vi "PT3_Create.vi"(5 "Save pt3":bool=TRUE, 7 "overwrite existing":bool, 8 "error in":errorcluster, 9 "Comment":string, 10 "pt3 header in":T1={"Comment"="", "RangeNo"=0, "Offset"=0, "AcquisitionTime (ms)"=0, "HardwareSerial"=0, "SyncDivider"=0, "Resolution (ns)"=0.0, "CFD Settings"={"Ch0 Level"=150, "Ch0 ZeroX"=10, "Ch1 Level"=50, "Ch1 ZeroX"=10}, "InpRate0"=0, "InpRate1"=0}, 11 "File Path":path) -> (0 "error out":errorcluster, 3 "refnum out":refnum<file>)   [LabVIEW 8.6]
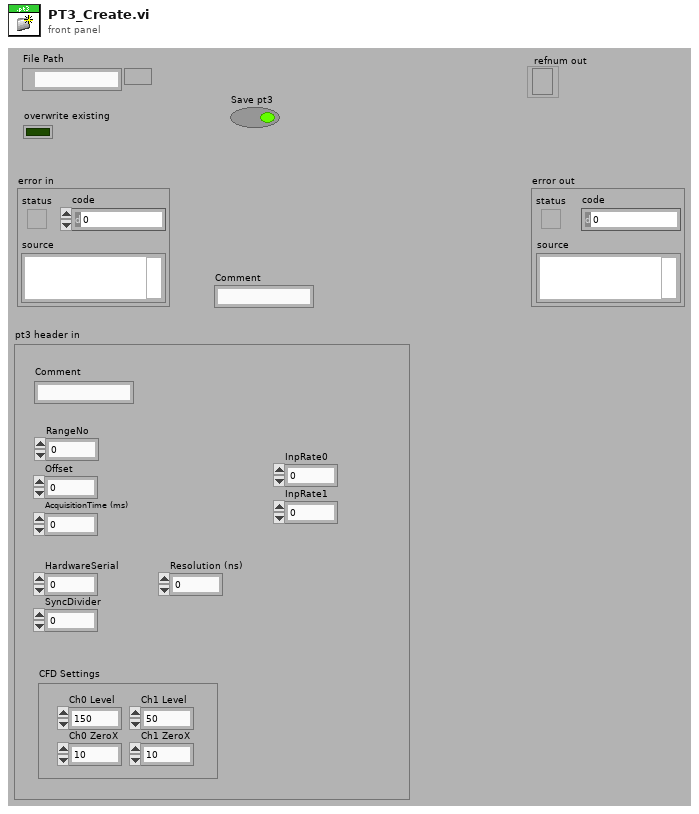
[diagram p1: front panel]
types:
  T1 = cluster{"Comment":string, "RangeNo":i32, "Offset":i32, "AcquisitionTime (ms)":i32, "HardwareSerial":i32, "SyncDivider":i32, "Resolution (ns)":sgl, "CFD Settings":cluster{"Ch0 Level":i32, "Ch0 ZeroX":i32, "Ch1 Level":i32, "Ch1 ZeroX":i32}, "InpRate0":i32, "InpRate1":i32}
  T2 = enum16{"big-endian, network order", "native, host order", "little-endian"}
  T3 = enum16{"open", "replace", "create", "open or create", "replace or create", "replace or create with confirmation"}
  T4 = cluster{"HardwareSerial":i32, "SyncDivider":i32, "Ch0 ZeroX":i32, "Ch0 Level":i32, "Ch1 ZeroX":i32, "Ch1 Level":i32, "Resolution (ns)":sgl, "RouterModelCode":i32, "RouterEnabled":i32}
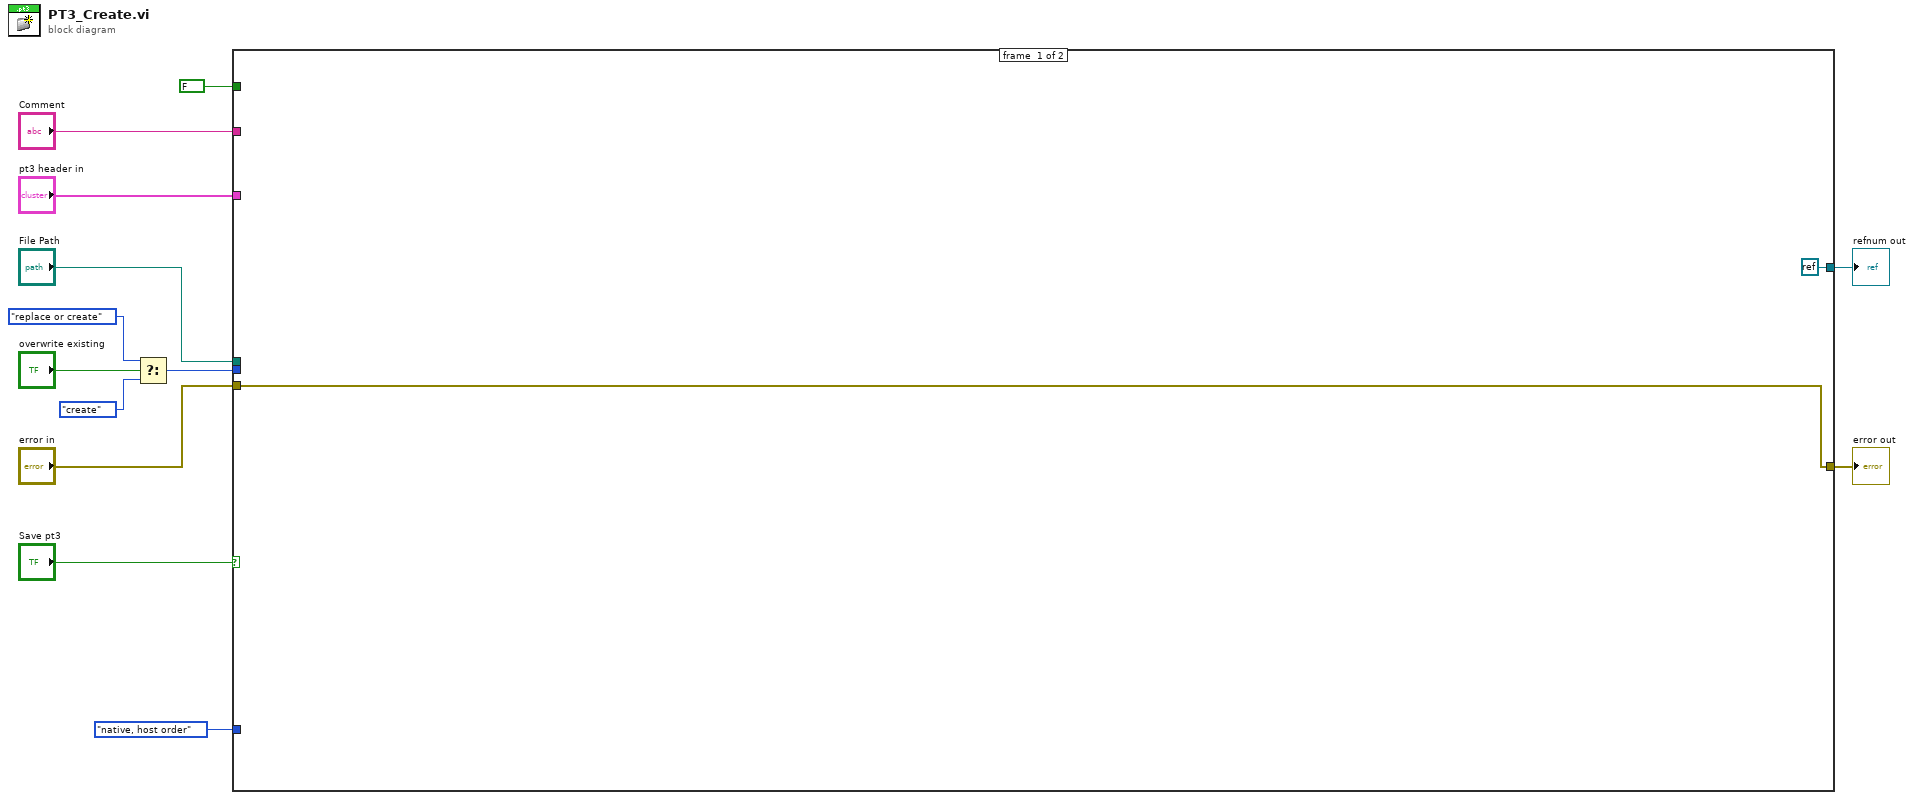
[diagram p0: block diagram]
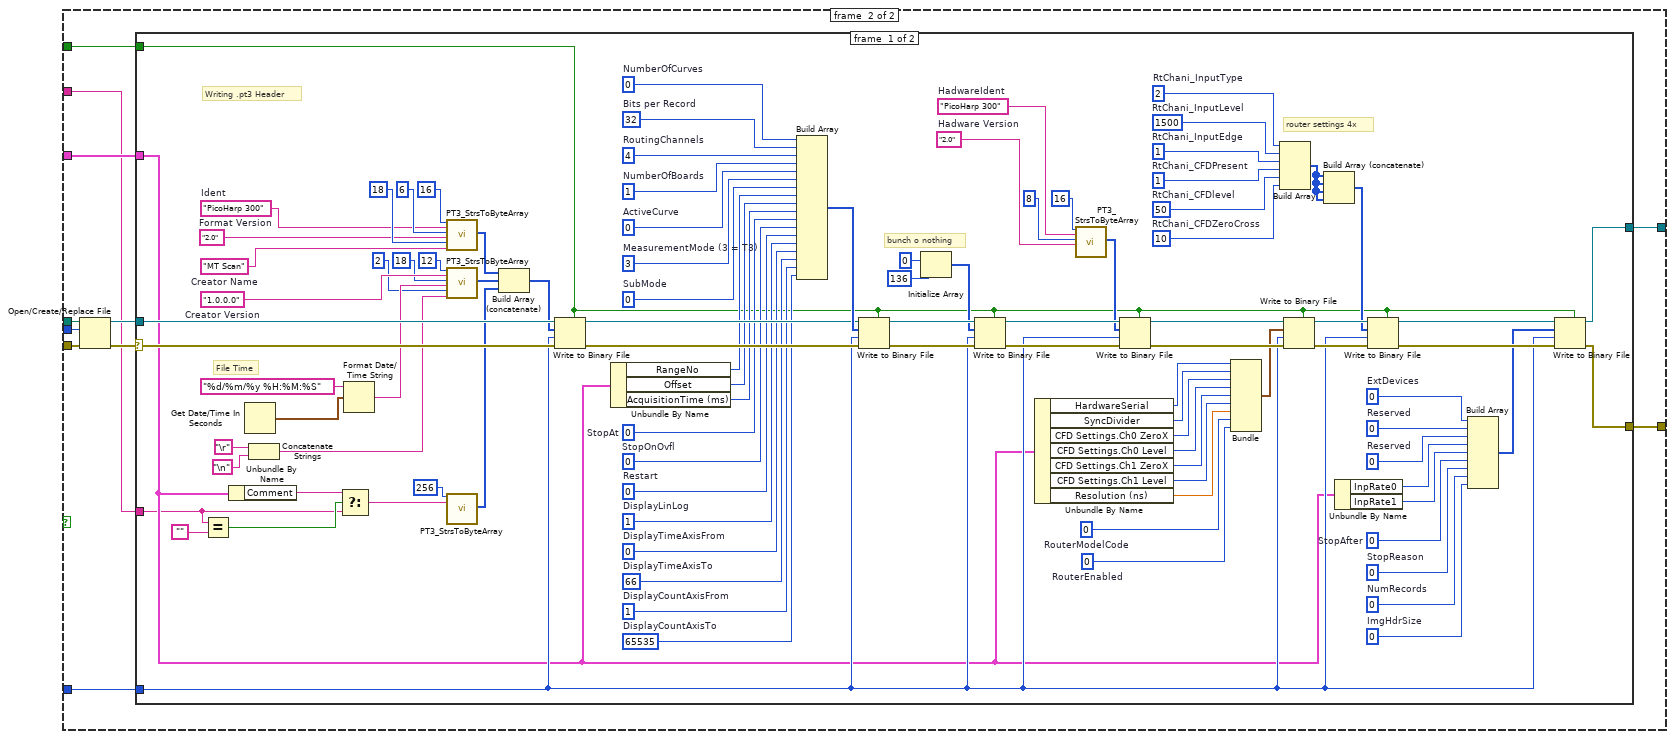
[diagram p2: hidden frame]
diagram:
  n1 = Select(t=T3."replace or create" ("operation (0:open)"), s="overwrite existing", f=T3."create" ("operation (0:open)")) -> (s? t:f=w9:T3)
  n2 = case shown="True" "Save pt3" {
    tunnel: "File Path" -> [_ w26]
    tunnel: w9 -> [_ w25]
    tunnel: "error in" -> [w15 w24]
    tunnel: [w15 w22] -> w7
    tunnel: [refnum<k0> refnum w20] -> w6
    tunnel: "pt3 header in" -> [_ w19]
    tunnel: T2."native, host order" ("byte order (0:big-endian, network order)") -> [_ w18]
    tunnel: FALSE ("prepend array or string size? (T)") -> [_ w17]
    tunnel: "Comment" -> [_ w16]
    frame #0 {
    }
    frame #1 {
      n3 = Open/Create/Replace File(file path (use dialog)=w26, error in=w24, operation (0:open)=w25) -> (refnum out=w21:refnum<file>, error out=w23:errorcluster)  [unwired: 4 out]
      n4 = case shown="No Error" w23 {
        selector: w23 -> [w126 w128]
        tunnel: [w34 w128] -> w22
        tunnel: w21 -> [w125 w127]
        tunnel: [w33 w127] -> w20
        tunnel: w19 -> [w45 _]
        tunnel: w18 -> [w46 _]
        tunnel: w17 -> [w47 _]
        tunnel: w16 -> [w28 _]
        frame #0 {
          w36 = 0  # ImgHdrSize
          w37 = 0  # NumRecords
          w38 = 0  # StopReason
          w39 = 0  # StopAfter
          w42 = 0  # Reserved
          w43 = 0  # Reserved
          w44 = 0  # ExtDevices
          w52 = 10  # RtChani_CFDZeroCross
          w54 = 50  # RtChani_CFDlevel
          w53 = 1  # RtChani_CFDPresent
          w55 = 1  # RtChani_InputEdge
          w56 = 1500  # RtChani_InputLevel
          w57 = 2  # RtChani_InputType
          w62 = 0  # RouterModelCode
          w61 = 0  # RouterEnabled
          w72 = "2.0"  # Hadware Version
          w74 = "PicoHarp 300"  # HadwareIdent
          w83 = 65535  # DisplayCountAxisTo
          w84 = 1  # DisplayCountAxisFrom
          w85 = 66  # DisplayTimeAxisTo
          w86 = 0  # DisplayTimeAxisFrom
          w87 = 1  # DisplayLinLog
          w88 = 0  # Restart
          w89 = 0  # StopOnOvfl
          w90 = 0  # StopAt
          w94 = 0  # SubMode
          w95 = 3  # MeasurementMode (3 = T3)
          w96 = 0  # ActiveCurve
          w97 = 1  # NumberOfBoards
          w98 = 4  # RoutingChannels
          w101 = 32  # Bits per Record
          w102 = 0  # NumberOfCurves
          w114 = "1.0.0.0"  # Creator Version
          w115 = "MT Scan"  # Creator Name
          w116 = "2.0"  # Format Version
          w117 = "PicoHarp 300"  # Ident
          # "router settings 4x"
          # "bunch o nothing"
          # "File Time"
          # "Writing .pt3 Header"
          n5 = Equal?(x=w28, y="") -> (x = y?=w30:bool)
          n6 = Unbundle By Name(w45) -> ("Comment"=w29:string)
          n7 = Get Date/Time In Seconds() -> (seconds since 1Jan1904=w122:timestamp)
          n8 = Concatenate Strings("\r", "\n") -> (w112:string)
          n9 = Select(t=w29, s=w30, f=w28) -> (s? t:f=w27:string)
          n10 = Format Date/Time String(time format string (%c)="%d/%m/%y %H:%M:%S", seconds (now)=w122) -> (date/time string=w113:string)  [unwired: 1 out]
          n11 = call "PT3_StrsToByteArray.vi"("Length"=16, "String"=w117, "Length 2"=6 ("Length"), "String 2"=w116, "Length 3"=18 ("Length"), "String 3"=w115) -> ("Byte Array"=w108:u8[])  [unwired: 1 in, 12 out]
          n12 = call "PT3_StrsToByteArray.vi"("Length"=12, "String"=w114, "Length 2"=18 ("Length"), "String 2"=w113, "Length 3"=2 ("Length"), "String 3"=w112) -> ("Byte Array"=w107:u8[])  [unwired: 1 in, 12 out]
          n13 = call "PT3_StrsToByteArray.vi"("Length"=256, "String"=w27) -> ("Byte Array"=w105:u8[])  [unwired: 5 in, 12 out]
          n14 = Build Array (concatenate)(w108, w107, w105) -> (w104:u8[])
          n15 = Write to Binary File(file (use dialog)=w125, data=w104, error in=w126, 5:w47, 9:w46) -> (refnum out=w99:refnum<file>, error out=w100:errorcluster)  [unwired: 2 out]
          n16 = Unbundle By Name(w45) -> ("RangeNo"=w93:i32, "Offset"=w92:i32, "AcquisitionTime (ms)"=w91:i32)
          n17 = Build Array(w102, w101, w98, w97, w96, w95, w94, w93, w92, w91, w90, w89, w88, w87, w86, w85, w84, w83) -> (w103:i32[])
          n18 = Write to Binary File(file (use dialog)=w99, data=w103, error in=w100, 5:w47, 9:w46) -> (refnum out=w81:refnum<file>, error out=w82:errorcluster)  [unwired: 2 out]
          n19 = Initialize Array(u8 0 ("element"), 136 ("dimension size")) -> (w78:u8[])
          n20 = Write to Binary File(file (use dialog)=w81, data=w78, error in=w82, 5:w47, 9:w46) -> (refnum out=w76:refnum<file>, error out=w77:errorcluster)  [unwired: 2 out]
          n21 = Unbundle By Name(w45) -> ("HardwareSerial"=w68:i32, "SyncDivider"=w67:i32, "CFD Settings.Ch0 ZeroX"=w66:i32, "CFD Settings.Ch0 Level"=w65:i32, "CFD Settings.Ch1 ZeroX"=w64:i32, "CFD Settings.Ch1 Level"=w63:i32, "Resolution (ns)"=w32:sgl)
          n22 = call "PT3_StrsToByteArray.vi"("Length"=16, "String"=w74, "Length 2"=8, "String 2"=w72) -> ("Byte Array"=w75:u8[])  [unwired: 3 in, 12 out]
          n23 = Write to Binary File(file (use dialog)=w76, data=w75, error in=w77, 5:w47, 9:w46) -> (refnum out=w69:refnum<file>, error out=w70:errorcluster)  [unwired: 2 out]
          n24 = Bundle("HardwareSerial"=w68, "SyncDivider"=w67, "Ch0 ZeroX"=w66, "Ch0 Level"=w65, "Ch1 ZeroX"=w64, "Ch1 Level"=w63, "Resolution (ns)"=w32, "RouterModelCode"=w62, "RouterEnabled"=w61) -> (w60:T4)  [unwired: 1 out]
          n25 = Build Array(w57, w56, w55, w53, w54, w52) -> (w51:i32[])
          n26 = Write to Binary File(file (use dialog)=w69, data=w60, error in=w70, 5:w47, 9:w46) -> (refnum out=w58:refnum<file>, error out=w59:errorcluster)  [unwired: 2 out]
          n27 = Build Array (concatenate)(w51, w51, w51, w51) -> (w50:i32[])
          n28 = Unbundle By Name(w45) -> ("InpRate0"=w41:i32, "InpRate1"=w40:i32)
          n29 = Write to Binary File(file (use dialog)=w58, data=w50, error in=w59, 5:w47, 9:w46) -> (refnum out=w48:refnum<file>, error out=w49:errorcluster)  [unwired: 2 out]
          n30 = Build Array(w44, w43, w42, w41, w40, w39, w38, w37, w36) -> (w35:i32[])
          n31 = Write to Binary File(file (use dialog)=w48, data=w35, error in=w49, 5:w47, 9:w46) -> (refnum out=w33:refnum<file>, error out=w34:errorcluster)  [unwired: 2 out]
        }
        frame #1 {
        }
      }
    }
  }
  "refnum out" <- w6
  "error out" <- w7
